vi "Start SECS.vi"(8 "error in":errorcluster) -> (0 "error out":errorcluster)   [LabVIEW 2020, in "SECS Bridge.lvlib"]
uses:
  SECS Bridge.lvlib
  Private/SECS Bridge Main.vi
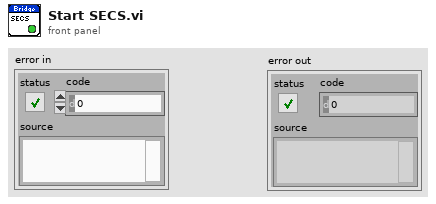
[diagram p1: front panel]
types:
  T1 = enum32{"Bad", "Idle", "Run top level", "Running"}
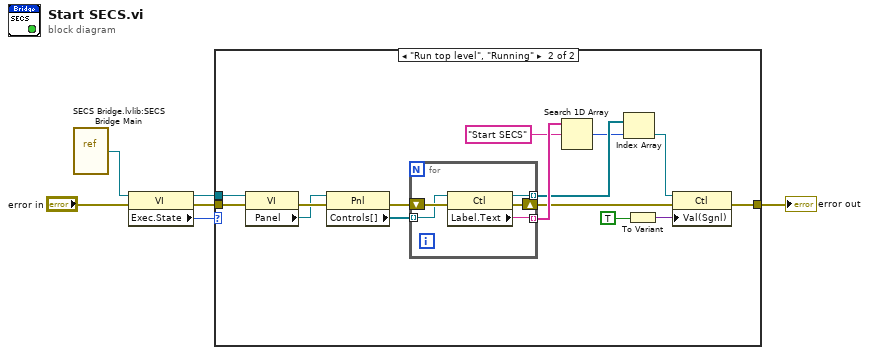
[diagram p0: block diagram]
diagram:
  n1 = vi-ref "SECS Bridge.lvlib:SECS Bridge Main.vi"() -> (w6:refnum<vi>)
  n2 = property class="VI"(reference=w6, error in="error in") -> (reference out=w2:refnum<vi>, error out=w3:errorcluster, "Exec.State"=w4:T1)
  n3 = case shown="\"Run top level\", \"Running\"" w4 {
    tunnel: w3 -> [w7 w22]
    tunnel: w2 -> [_ w21]
    tunnel: [w7 w8] -> w1
    frame Default {
    }
    frame "Run top level", "Running" {
      n4 = property class="VI"(reference=w21, error in=w22) -> (error out=w20:errorcluster, "Panel"=w19:refnum<vi>)  [unwired: 1 out]
      n5 = property class="Pnl"(reference=w19, error in=w20) -> (error out=w17:errorcluster, "Controls[]"=w18:refnum<vi>[])  [unwired: 1 out]
      n6 = for {
        tunnel: w18 -> [w26] mode=indexing
        shift-right: [w25] -> w12
        shift-left: w17 -> [w27]
        tunnel: [w24] -> w14 mode=indexing
        tunnel: [w23] -> w16 mode=indexing
        n7 = property class="Ctl"(reference=w26, error in=w27) -> (reference out=w24:refnum<vi>, error out=w25:errorcluster, "Label.Text"=w23:string)
      }
      n8 = Search 1D Array(1D array=w16, element="Start SECS") -> (index of element=w13:i32)  [unwired: 1 in]
      n9 = Index Array(array=w14, index=w13) -> (element=w11:refnum<vi>)
      n10 = To Variant(anything=TRUE) -> (Variant=w10:variant)
      n11 = property class="Ctl"(reference=w11, error in=w12, "Val(Sgnl)"=w10) -> (error out=w8:errorcluster)  [unwired: 1 out]
    }
  }
  "error out" <- w1
